vi "Release.vi"(8 "Error In":errorcluster, 11 "Tree Data":refnum<class "Tree Data.lvclass">) -> (0 "Error Out":errorcluster)   [LabVIEW 2017, in "Tree API.lvlib" / "Tree Data.lvclass"]
doc: "This is an abstract method defining an interface for Tree Data Release functionality, invoked in the Tree API with Delete methods. Override it in child classes."
uses:
  Tree Data.lvclass
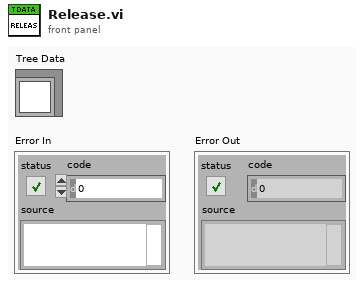
[diagram p1: front panel]
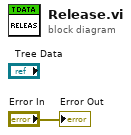
[diagram p0: block diagram]
diagram:
  "Error Out" <- "Error In"
